vi "Initialize.vi"(8 "error in (no error)":errorcluster, 11 "Device Item Ref in":T1 format="%.0x") -> (0 "error out":errorcluster, 3 "Device Item Ref out":T1 format="%.0x")   [LabVIEW 2020, in "Communication Bus Template System Explorer.lvlib" / "Implementation.lvlib"]
uses:
  Implementation.lvlib
  <vilib>/NI VeriStand/Custom Device API/Custom Device Item Ref.ctl
  <vilib>/NI/NI VeriStand Custom Device Import and Export Tool/ImportExport.lvlib
  Scripting/Communication Bus Template Scripting.lvlib
  <vilib>/NI VeriStand/Custom Device API/Custom Device API.lvlib
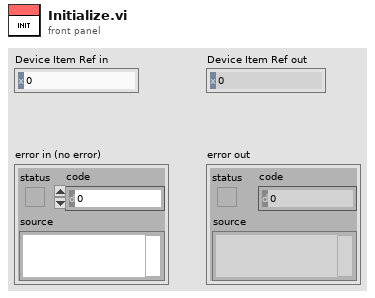
[diagram p1: front panel]
types:
  T1 = typedef "Custom Device API.lvlib/Custom Device Item Ref.ctl" = u64
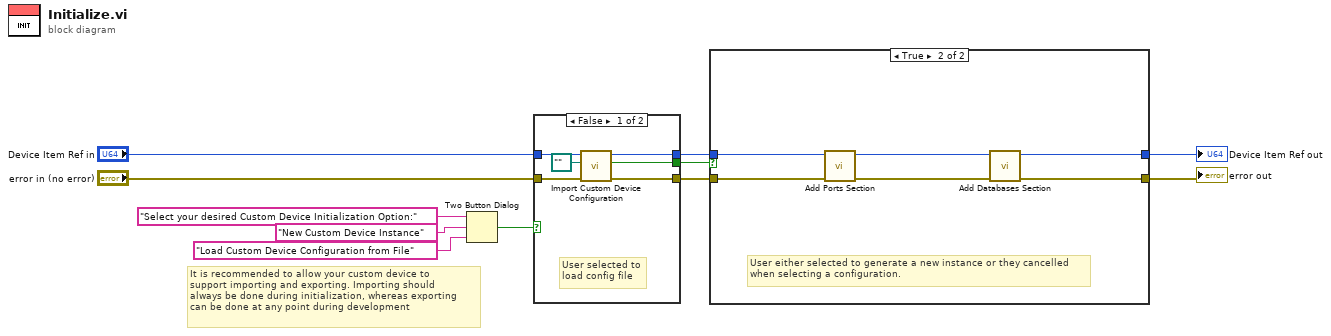
[diagram p0: block diagram]
diagram:
  # "It is recommended to allow your custom device to\nsupport importing and exporting. Importing should\nalways be done during initialization, whereas exporting\ncan be done at any point during development"
  n1 = Two Button Dialog(message="Select your desired Custom Device Initialization Option:", 1:"Load Custom Device Configuration from File" ("F button name (\"Cancel\")"), 2:"New Custom Device Instance" ("T button name (\"OK\")")) -> (T button?=w8:bool)
  n2 = case shown="False" w8 {
    selector: w8 -> [_ w18]
    tunnel: "Device Item Ref in" -> [w17 w20]
    tunnel: [w16 w20] -> w7
    tunnel: "error in (no error)" -> [w14 w19]
    tunnel: [w13 w19] -> w5
    tunnel: [w12 w18] -> w6
    frame False {
      # "User selected to\nload config file"
      n3 = call <vilib>:"Import Custom Device Configuration.vi"("error in (no error)"=w14, "Path"=path "", "NodeID"=w17) -> ("error out"=w13:errorcluster, "cancelled"=w12:bool, "NodeID out"=w16:u64)  [unwired: 6 in]
    }
    frame True {
      # "User selected new\ncustom device. Do\nnothing in this case\nand handle new\ngeneration in the\nnext case structure"
    }
  }
  n4 = case shown="True" w6 {
    tunnel: w7 -> [w22 w27]
    tunnel: w5 -> [w21 w28]
    tunnel: [w21 w24] -> w1
    tunnel: [w22 w23] -> w2
    frame False {
      # "User selected to import from configuration and didn't cancel import"
    }
    frame True {
      # "User either selected to generate a new instance or they cancelled\nwhen selecting a configuration."
      n5 = call "Add Ports Section.vi"("error in"=w28, "Custom device Ref"=w27) -> ("error out"=w25:errorcluster, "Custom device Ref out"=w26:T1)  [unwired: 8 in]
      n6 = call "Add Databases Section.vi"("error in"=w25, "Custom device Ref"=w26) -> ("error out"=w24:errorcluster, "Custom device Ref out"=w23:T1)  [unwired: 8 in]
    }
  }
  "error out" <- w1
  "Device Item Ref out" <- w2
